vi "PXI-Check For Abort.vi"(0 "error in (no error)":errorcluster, 12 "DAQ Write State":T1) -> (4 "error out":errorcluster, 8 "Ramping":T2, 14 "DAQ Write State Out":T1, 15 "Zero?":bool)   [LabVIEW 2020]
uses:
  Type Defs/Ramping Params.ctl
  Type Defs/DAQ Write State enum.ctl
  PXI Globals.vi
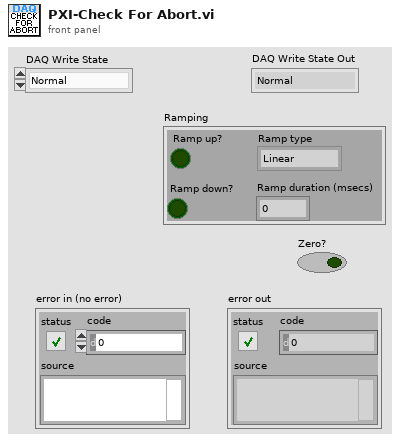
[diagram p1: front panel]
types:
  T1 = typedef "DAQ Write State enum.ctl" = enum16{"Normal", "Ramp down", "Zero buffers", "Done"}
  T2 = typedef "Ramping Params.ctl" = cluster{"Ramp up?":bool, "Ramp down?":bool, "Ramp duration (msecs)":dbl, "Ramp type":enum16{"Linear", "Cos2"}}
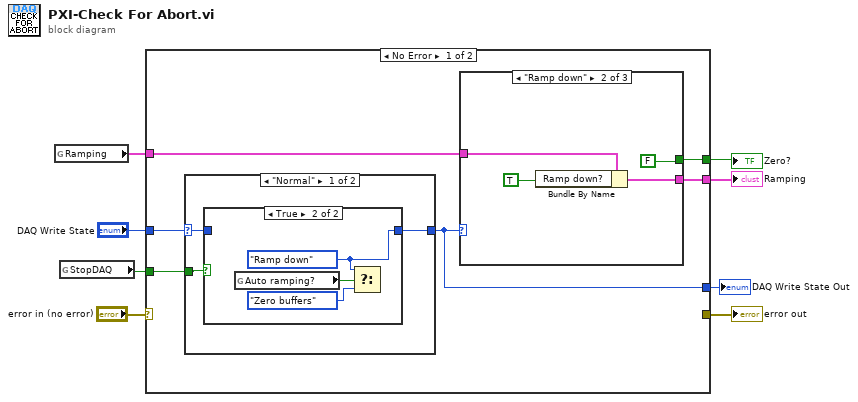
[diagram p0: block diagram]
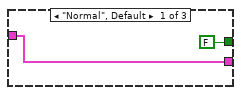
[diagram p4: hidden frame]
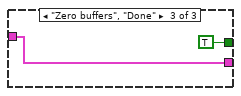
[diagram p5: hidden frame]
diagram:
  n1 = global read "PXI Globals.vi" "Ramping"() -> (w5:T2)
  n2 = global read "PXI Globals.vi" "StopDAQ"() -> (w2:bool)
  n3 = case shown="No Error" "error in (no error)" {
    selector: "error in (no error)" -> [_ w32]
    tunnel: [w14 _] -> w8
    tunnel: "DAQ Write State" -> [w10 w31]
    tunnel: [w13 _] -> w6
    tunnel: w5 -> [w12 _]
    tunnel: [_ w32] -> w3
    tunnel: w2 -> [w11 _]
    tunnel: [w9 w31] -> w1
    frame No Error {
      n4 = case shown="\"Normal\"" w10 {
        selector: w10 -> [w15 w22]
        tunnel: w11 -> [w17 _]
        tunnel: [w16 w22] -> w9
        frame "Normal" {
          n5 = case shown="True" w17 {
            tunnel: [w18 w19] -> w16
            tunnel: w15 -> [w18 _]
            frame False {
            }
            frame True {
              w19 = DAQ_Write_State_enum."Ramp down" ("t")
              n6 = global read "PXI Globals.vi" "Auto ramping?"() -> (w21:bool)
              n7 = Select(t=w19, s=w21, f=DAQ_Write_State_enum."Zero buffers") -> ()  [unwired: 1 out]
            }
          }
        }
        frame "Ramp down", Default {
        }
      }
      n8 = case shown="\"Ramp down\"" w9 {
        tunnel: w12 -> [w23 w28 w29]
        tunnel: [FALSE FALSE TRUE] -> w13
        tunnel: [w23 w25 w29] -> w14
        frame "Normal", Default {
        }
        frame "Ramp down" {
          n9 = Bundle By Name(cluster=w28, "Ramp down?"=TRUE) -> (w25:T2)
        }
        frame "Zero buffers", "Done" {
        }
      }
    }
    frame Error {
    }
  }
  "Ramping" <- w8
  "Zero?" <- w6
  "error out" <- w3
  "DAQ Write State Out" <- w1
